vi "Write Sub Panel Paquetes 1.vi"(8 "error in (no error)":errorcluster, 10 "Sub Panel Paquetes":refnum<vi>, 11 "Paquetes in":refnum<class "Paquetes.lvclass">) -> (0 "error out":errorcluster, 3 "Paquetes out":refnum<class "Paquetes.lvclass">)   [LabVIEW 2020, in "Paquetes.lvlib" / "Paquetes.lvclass"]
uses:
  Paquetes.lvclass
  Paquetes.lvclass/Paquetes.ctl
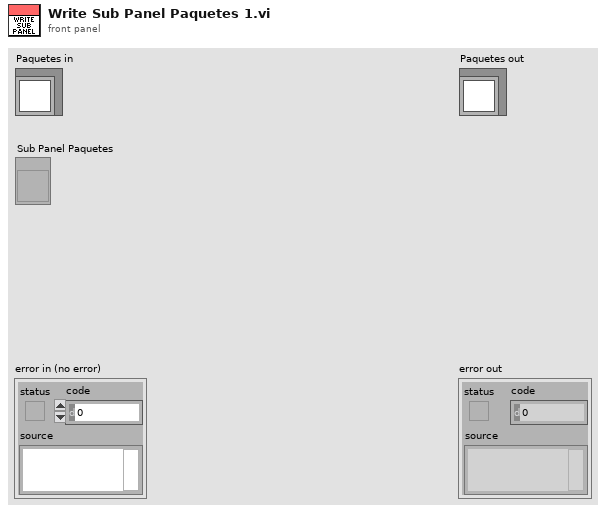
[diagram p1: front panel]
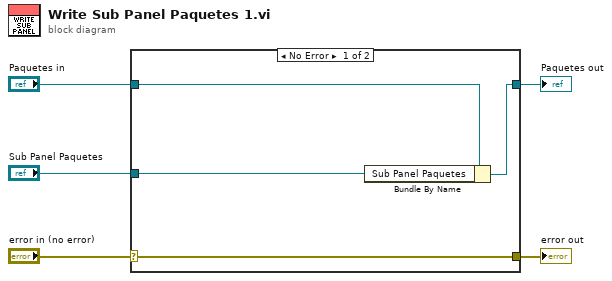
[diagram p0: block diagram]
diagram:
  n1 = case shown="No Error" "error in (no error)" {
    selector: "error in (no error)" -> [w9 w10]
    tunnel: [w9 w10] -> w4
    tunnel: [w7 w11] -> w2
    tunnel: "Paquetes in" -> [w8 w11]
    tunnel: "Sub Panel Paquetes" -> [w6 _]
    frame No Error {
      n2 = Bundle By Name(cluster=w8, "Sub Panel Paquetes"=w6) -> (w7:refnum<class "Paquetes.lvclass">)
    }
    frame Error {
    }
  }
  "error out" <- w4
  "Paquetes out" <- w2
